vi "Write DVR_voltage.vi"(8 "error in (no error)":errorcluster, 10 "DVR_voltage":refnum<data-value>, 11 "DAQ Voltage in":refnum<class "DAQ Voltage.lvclass">) -> (0 "error out":errorcluster, 3 "DAQ Voltage out":refnum<class "DAQ Voltage.lvclass">)   [LabVIEW 2025, in "DAQ Voltage.lvlib" / "DAQ Voltage.lvclass"]
uses:
  DAQ Voltage.lvclass
  DAQ Voltage.lvclass/DAQ Voltage.ctl
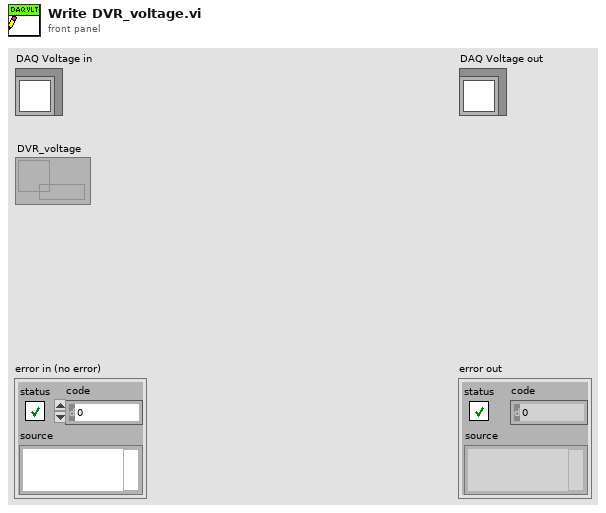
[diagram p1: front panel]
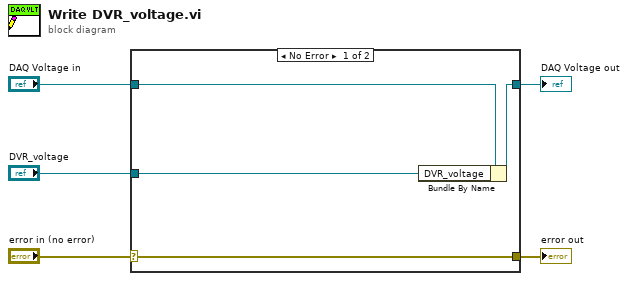
[diagram p0: block diagram]
diagram:
  n1 = case shown="No Error" "error in (no error)" {
    selector: "error in (no error)" -> [w9 w10]
    tunnel: [w9 w10] -> w4
    tunnel: [w7 w11] -> w2
    tunnel: "DAQ Voltage in" -> [w8 w11]
    tunnel: "DVR_voltage" -> [w6 _]
    frame No Error {
      n2 = Bundle By Name(cluster=w8, "DVR_voltage"=w6) -> (w7:refnum<class "DAQ Voltage.lvclass">)
    }
    frame Error {
    }
  }
  "error out" <- w4
  "DAQ Voltage out" <- w2
